vi "DAQmx_AD+FFT(連續採樣).vi"() -> ()   [LabVIEW 2010]
uses:
  <vilib>/DAQmx/create/channels.llb/DAQmx Create Channel (AI-Voltage-Basic).vi
  <vilib>/DAQmx/configure/timing.llb/DAQmx Timing (Sample Clock).vi
  <vilib>/Utility/error.llb/DialogType.ctl
  <vilib>/DAQmx/read.llb/DAQmx Read (Analog 1D DBL 1Chan NSamp).vi
  <vilib>/measure/NI_MAPro.lvlib
  <vilib>/measure/maspectr.llb/FFT Spectrum (Mag-Phase) for 1 Chan.vi
panel:
  out "FFT":cluster{"f0":dbl, "df":dbl, "magnitude":dbl[]}(graph)
  out "time":dbl[](graph)
  out "迴圈數":i32
  in  "stop":bool
  out "message":string=" INSTRUCTIONS:\r\rNormal Use:  When using subVIs that incorporate the error in/error out (or error I/O) structure, place this handler where you want to inform the user of an error, typically at the end of the I/O data path, as the last action of the program.  If the error in error? is ERROR, the handler creates a message describing the error and its source.  If the type of dialog = 1 (default), the message is displayed to the user, who can only acknowedge it.  If the type = 2, the user can acknowledge the message or abort execution; aborting a program with active I/O is not recommended.  If the type = 0, no message is displayed; this is used to process the error programmatically, and the error out cluster elements are wired to individual terminals for that reason.  \r\rOther Use:\n\r\nlocal testing.  To test the error code of a subVI or function that does not have the error I/O structure, you can wire its error code and a source string to the local error code and error source inputs.  If error in error? indicates no error and error code is not equal to 0, the local code and source are substituted for the error in values, and error? is set TRUE (ERROR)."
  in  "samples per channel(設定Buffer數)":i32=1000
  in  "sample mode(取樣模式)":i32(ring)=10123 items=["Finite Samples"=10178, "Continuous Samples"=10123, "Hardware Timed Single Point"=12522]
  in  "rate(取樣頻率)":dbl=1000.0 format="%0.2f"
  in  "physical channels":tag="PCI-6035E/ai0"
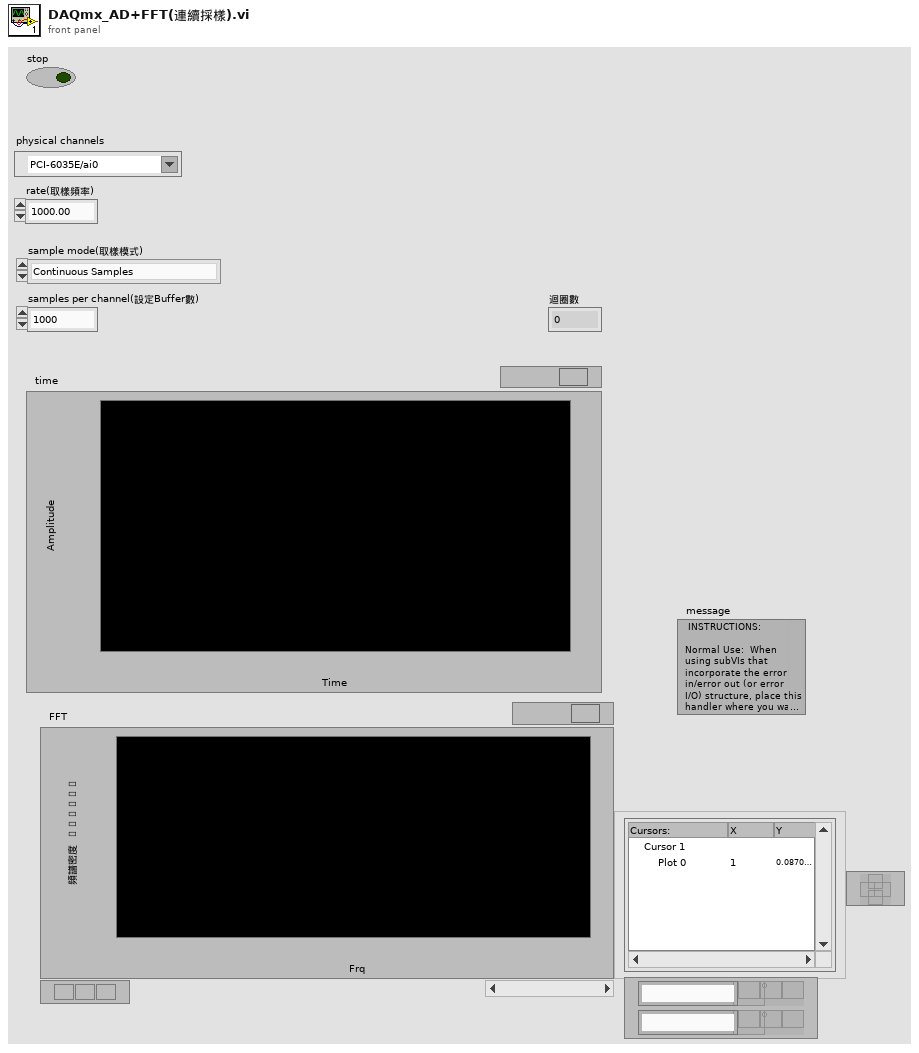
[diagram p1: front panel]
types:
  T1 = typedef "DialogType.ctl" = u16
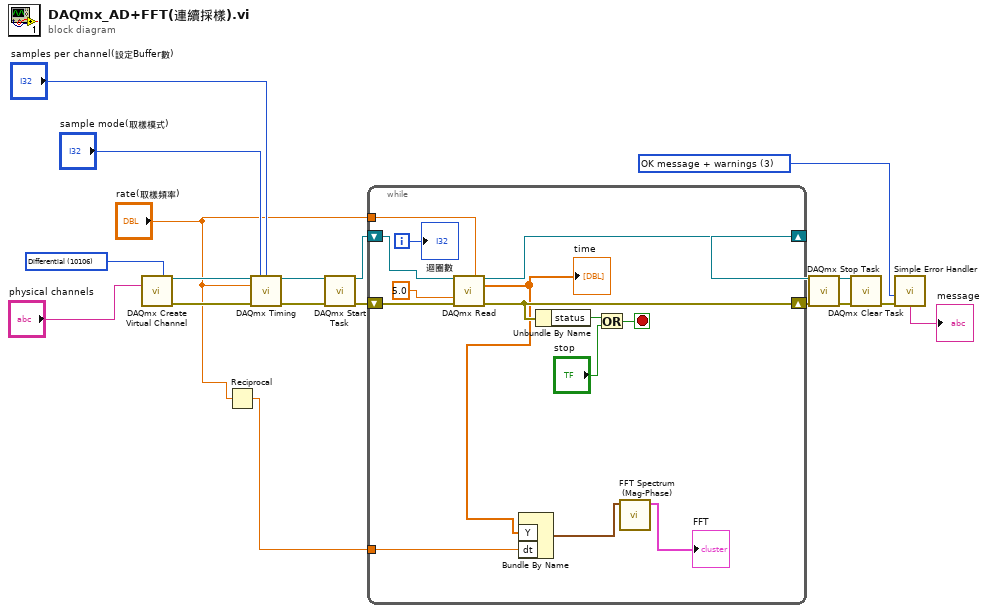
[diagram p0: block diagram]
diagram:
  w6 = T1 3 items=["no dialog", "OK message", "continue or stop message", "OK message + warnings", "continue/stop + warnings"] ("type of dialog (OK msg:1)")
  w18 = 10106 items=["Default"=-1, "RSE"=10083, "NRSE"=10078, "Differential"=10106, "Pseudodifferential"=12529] ("input terminal configuration")
  n1 = call-poly <vilib>:"DAQmx Create Virtual Channel.vi"("input terminal configuration"=w18, "physical channels"="physical channels") -> ("task out"=w17:refnum<k21>, "error out"=w12:errorcluster)  [unwired: 12 in]
  n2 = Reciprocal(x="rate(取樣頻率)") -> (1/x=w2:dbl)
  n3 = call-poly <vilib>:"DAQmx Timing.vi"("task/channels in"=w17, "sample mode"="sample mode(取樣模式)", "samples per channel"="samples per channel(設定Buffer數)", "rate"="rate(取樣頻率)", "error in"=w12) -> ("task out"=w4:refnum<k21>, "error out"=w3:errorcluster)  [unwired: 9 in]
  n4 = call <vilib>:"DAQmx Start Task.vi"("task/channels in"=w4, "error in"=w3) -> ("task out"=w16:refnum<k21>, "error out"=w11:errorcluster)  [unwired: 12 in]
  n5 = while {
    shift-right: [w32] -> w15
    shift-left: w16 -> [w33]
    shift-right: [w29] -> w10
    shift-left: w11 -> [w31]
    tunnel: w2 -> [w21]
    tunnel: "rate(取樣頻率)" -> [w20]
    i -> [w28]
    stop <- w25 stop-if-true
    n6 = call-poly <vilib>:"DAQmx Read.vi"("task/channels in"=w33, "number of samples per channel"=w20, "timeout"=5.0, "error in"=w31) -> ("task out"=w32:refnum<k21>, "data"=w24:dbl[], "error out"=w29:errorcluster)  [unwired: 9 in]
    "time" <- w24
    n7 = Bundle By Name("Y"=w24, "dt"=w21) -> (w23:waveform(dbl))  [unwired: 1 in]
    n8 = Unbundle By Name(w29) -> ("status"=w26:bool)
    n9 = Or(x=w26, y="stop") -> (x .or. y?=w25:bool)
    n10 = call-poly <vilib>:"FFT Spectrum (Mag-Phase).vi"("time signal"=w23) -> ("magnitude"=→"FFT":cluster{"f0":dbl, "df":dbl, "magnitude":dbl[]})  [unwired: 6 in, 4 out]
    "迴圈數" <- w28
  }
  n11 = call <vilib>:"DAQmx Stop Task.vi"("task/channels in"=w15, "error in"=w10) -> ("task out"=w14:refnum<k21>, "error out"=w9:errorcluster)  [unwired: 12 in]
  n12 = call <vilib>:"DAQmx Clear Task.vi"("task in"=w14, "error in"=w9) -> ("error out"=w13:errorcluster)  [unwired: 13 in]
  n13 = call <vilib>:"Simple Error Handler.vi"("type of dialog (OK msg:1)"=w6, "error in (no error)"=w13) -> ("message"=→"message":string)  [unwired: 3 in, 4 out]
